vi "QFT-4Q.vi"   [LabVIEW 2020]
uses:
  QuSim/QuVI_Wire (initial).vi
  QuSim/QuVI_Wire (added).vi
  Gates/Polymorphs/Pauli-Z_s.vi
  Gates/Polymorphs/^Control_e.vi
  Gates/Polymorphs/vSwap_e.vi
  Gates/Polymorphs/^Swap_e.vi
  Analysis/Inspect VIs/Probability Bar.vi
panel:
  # "Quantum Fourier Transform Example"
  # "*Open the block diagram for the circuit view (Ctrl+E)"
  # "Demonstrates the Quantum Fourier Transform (QFT) on a 4-qubit register.\n\nThis example implements the QFT algorithm, which transforms a quantum state from the computational basis to the Fourier basis. It applies a sequence of Hadamard gates and controlled-rotation gates to encode the amplitudes' frequency information into the phases. Run this VI to see how periodic states are transformed."
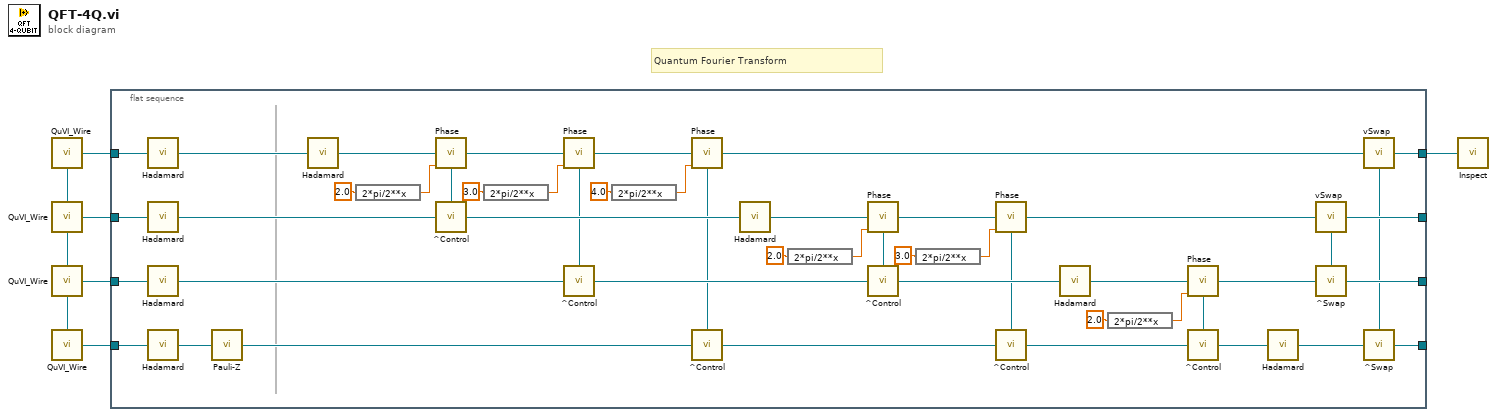
[diagram p0: block diagram]
diagram:
  # "Quantum Fourier Transform"
  n1 = call-poly "QuVI_Wire.vi"() -> ("QuWire out"=w6:refnum<class "QuWire.lvclass">, "Stack out"=w8:refnum<class "QuSim.lvclass">)  [unwired: 14 in]
  n2 = call-poly "QuVI_Wire.vi"("Stack in"=w8) -> ("QuWire out"=w7:refnum<class "QuWire.lvclass">, "Stack out"=w4:refnum<class "QuSim.lvclass">)  [unwired: 13 in]
  n3 = call-poly "QuVI_Wire.vi"("Stack in"=w4) -> ("QuWire out"=w5:refnum<class "QuWire.lvclass">, "Stack out"=w2:refnum<class "QuSim.lvclass">)  [unwired: 13 in]
  n4 = call-poly "QuVI_Wire.vi"("Stack in"=w2) -> ("QuWire out"=w3:refnum<class "QuWire.lvclass">)  [unwired: 13 in, 1 out]
  n5 = flat-sequence {
    tunnel: w7 -> [w56]
    tunnel: w6 -> [w57]
    tunnel: w5 -> [w55]
    tunnel: w3 -> [w54]
    tunnel: [w12] -> w1
    tunnel: [w15] -> _
    tunnel: [w14] -> _
    tunnel: [w11] -> _
    frame #0 {
      n6 = call "Hadamard.vi"("QuWire in"=w57) -> ("QuWire out"=w52:refnum<class "QuWire.lvclass">)  [unwired: 14 in]
      n7 = call "Hadamard.vi"("QuWire in"=w56) -> ("QuWire out"=w49:refnum<class "QuWire.lvclass">)  [unwired: 14 in]
      n8 = call "Hadamard.vi"("QuWire in"=w55) -> ("QuWire out"=w53:refnum<class "QuWire.lvclass">)  [unwired: 14 in]
      n9 = call "Hadamard.vi"("QuWire in"=w54) -> ("QuWire out"=w51:refnum<class "QuWire.lvclass">)  [unwired: 14 in]
      n10 = call-poly "Pauli-Z.vi"("QuWire in"=w51) -> ("QuWire out"=w50:refnum<class "QuWire.lvclass">)  [unwired: 14 in]
      n11 = call "Hadamard.vi"("QuWire in"=w52) -> ("QuWire out"=w48:refnum<class "QuWire.lvclass">)  [unwired: 14 in]
      n12 = expression code="2*pi/2**x"(2.0) -> (w29:dbl)
      n13 = call-poly "^Control.vi"("QuWire in"=w49) -> ("^ Ctrl out"=w31:refnum<class "CtrlLine.lvclass">, "QuWire out"=w46:refnum<class "QuWire.lvclass">)  [unwired: 13 in]
      n14 = call "Phase.vi"("QuWire in"=w48, "phi"=w29, "^ Ctrl in"=w31) -> ("QuWire out"=w32:refnum<class "QuWire.lvclass">)  [unwired: 12 in]
      n15 = expression code="2*pi/2**x"(3.0) -> (w27:dbl)
      n16 = call-poly "^Control.vi"("QuWire in"=w53) -> ("^ Ctrl out"=w33:refnum<class "CtrlLine.lvclass">, "QuWire out"=w45:refnum<class "QuWire.lvclass">)  [unwired: 13 in]
      n17 = call "Phase.vi"("QuWire in"=w32, "phi"=w27, "^ Ctrl in"=w33) -> ("QuWire out"=w34:refnum<class "QuWire.lvclass">)  [unwired: 12 in]
      n18 = expression code="2*pi/2**x"(4.0) -> (w25:dbl)
      n19 = call-poly "^Control.vi"("QuWire in"=w50) -> ("^ Ctrl out"=w41:refnum<class "CtrlLine.lvclass">, "QuWire out"=w44:refnum<class "QuWire.lvclass">)  [unwired: 13 in]
      n20 = call "Phase.vi"("QuWire in"=w34, "phi"=w25, "^ Ctrl in"=w41) -> ("QuWire out"=w13:refnum<class "QuWire.lvclass">)  [unwired: 12 in]
      n21 = call "Hadamard.vi"("QuWire in"=w46) -> ("QuWire out"=w39:refnum<class "QuWire.lvclass">)  [unwired: 14 in]
      n22 = expression code="2*pi/2**x"(2.0) -> (w23:dbl)
      n23 = call-poly "^Control.vi"("QuWire in"=w45) -> ("^ Ctrl out"=w38:refnum<class "CtrlLine.lvclass">, "QuWire out"=w43:refnum<class "QuWire.lvclass">)  [unwired: 13 in]
      n24 = call "Phase.vi"("QuWire in"=w39, "phi"=w23, "^ Ctrl in"=w38) -> ("QuWire out"=w40:refnum<class "QuWire.lvclass">)  [unwired: 12 in]
      n25 = expression code="2*pi/2**x"(3.0) -> (w21:dbl)
      n26 = call-poly "^Control.vi"("QuWire in"=w44) -> ("^ Ctrl out"=w37:refnum<class "CtrlLine.lvclass">, "QuWire out"=w42:refnum<class "QuWire.lvclass">)  [unwired: 13 in]
      n27 = call "Phase.vi"("QuWire in"=w40, "phi"=w21, "^ Ctrl in"=w37) -> ("QuWire out"=w18:refnum<class "QuWire.lvclass">)  [unwired: 12 in]
      n28 = call "Hadamard.vi"("QuWire in"=w43) -> ("QuWire out"=w36:refnum<class "QuWire.lvclass">)  [unwired: 14 in]
      n29 = expression code="2*pi/2**x"(2.0) -> (w19:dbl)
      n30 = call-poly "^Control.vi"("QuWire in"=w42) -> ("^ Ctrl out"=w35:refnum<class "CtrlLine.lvclass">, "QuWire out"=w47:refnum<class "QuWire.lvclass">)  [unwired: 13 in]
      n31 = call "Phase.vi"("QuWire in"=w36, "phi"=w19, "^ Ctrl in"=w35) -> ("QuWire out"=w17:refnum<class "QuWire.lvclass">)  [unwired: 12 in]
      n32 = call "Hadamard.vi"("QuWire in"=w47) -> ("QuWire out"=w16:refnum<class "QuWire.lvclass">)  [unwired: 14 in]
      n33 = call-poly "vSwap.vi"("QuWire in"=w18) -> ("QuWire out"=w11:refnum<class "QuWire.lvclass">, "v Swap out"=w10:refnum<class "CtrlLine.lvclass">)  [unwired: 13 in]
      n34 = call-poly "^Swap.vi"("^ Swap in"=w10, "QuWire in"=w17) -> ("QuWire out"=w15:refnum<class "QuWire.lvclass">)  [unwired: 13 in]
      n35 = call-poly "vSwap.vi"("QuWire in"=w13) -> ("QuWire out"=w12:refnum<class "QuWire.lvclass">, "v Swap out"=w9:refnum<class "CtrlLine.lvclass">)  [unwired: 13 in]
      n36 = call-poly "^Swap.vi"("^ Swap in"=w9, "QuWire in"=w16) -> ("QuWire out"=w14:refnum<class "QuWire.lvclass">)  [unwired: 13 in]
    }
  }
  n37 = call-poly "Inspect.vi"("QuWire in"=w1) -> ()  [unwired: 15 in]
